vi "_nevstop_choosingDlg.vi"(8 "error in (no error)":errorcluster) -> (0 "error out":errorcluster, 1 "Cancelled?":bool=TRUE, 2 "QuckDrop":string, 3 "QDKS Info":T2[](array[typedef])=[{"VI Name"="Cluster AutoSizing", "VI Path"=path "C:/Program Files (x86)/National Instruments/LabVIEW 2014/resource/dialog/QuickDrop/plugins/QD_Cluster AutoSizing/Cluster AutoSizing.vi", "Default Shortcut"="U", "Assigned Shortcut"="u", "Description"="Using a float dialog to choose cluster auto-sizing type. Press `Shift` to set the contained cluster items recursively. \n\n- None\n- Size to Fit\n- Arrange Horizontally\n- Arrange Vertically\n\nDefault Shortcut - [U]"}, {"VI Name"="Align - Bottom Edges", "VI Path"=path "C:/Program Files (x86)/National Instruments/LabVIEW 2014/resource/dialog/QuickDrop/plugins/QD_Align&Distribute/Align - Bottom Edges.vi", "Default Shortcut"="v", "Assigned Shortcut"="v", "Description"="Align - Bottom Edges.vi\n"}, {"VI Name"="Align - Horizontal Centers", "VI Path"=path "C:/Program Files (x86)/National Instruments/LabVIEW 2014/resource/dialog/QuickDrop/plugins/QD_Align&Distribute/Align - Horizontal Centers.vi", "Default Shortcut"="v", "Assigned Shortcut"="", "Description"="Align - Horizontal Centers.vi"}, {"VI Name"="Align - Left Edges", "VI Path"=path "C:/Program Files (x86)/National Instruments/LabVIEW 2014/resource/dialog/QuickDrop/plugins/QD_Align&Distribute/Align - Left Edges.vi", "Default Shortcut"="v", "Assigned Shortcut"="5", "Description"="Align - Left Edges.vi"}, {"VI Name"="Align - Right Edges", "VI Path"=path "C:/Program Files (x86)/National Instruments/LabVIEW 2014/resource/dialog/QuickDrop/plugins/QD_Align&Distribute/Align - Right Edges.vi", "Default Shortcut"="v", "Assigned Shortcut"="", "Description"="Align - Right Edges.vi"}, {"VI Name"="Align - Top Edges", "VI Path"=path "C:/Program Files (x86)/National Instruments/LabVIEW 2014/resource/dialog/QuickDrop/plugins/QD_Align&Distribute/Align - Top Edges.vi", "Default Shortcut"="v", "Assigned Shortcut"="", "Description"="Align - Top Edges.vi"}, {"VI Name"="Align - Vertical Centers", "VI Path"=path "C:/Program Files (x86)/National Instruments/LabVIEW 2014/resource/dialog/QuickDrop/plugins/QD_Align&Distribute/Align - Vertical Centers.vi", "Default Shortcut"="v", "Assigned Shortcut"="", "Description"="Align - Vertical Centers.vi"}, {"VI Name"="Align and Distribute", "VI Path"=path "C:/Program Files (x86)/National Instruments/LabVIEW 2014/resource/dialog/QuickDrop/plugins/QD_Align&Distribute/Align and Distribute.vi", "Default Shortcut"="A", "Assigned Shortcut"="a", "Description"="Aligns selected items to the right, left, top or bottom or by horizontal or vertical centers by pressing r, l, t, b, h or v."}, {"VI Name"="Arrange VI Window", "VI Path"=path "C:/Program Files (x86)/National Instruments/LabVIEW 2014/resource/dialog/QuickDrop/plugins/QD_Arrange VI Window/Arrange VI Window.vi", "Default Shortcut"="F", "Assigned Shortcut"="f", "Description"="When used on the front panel:\n-Arranges controls and indicators to be consistent with the connector pane arrangement. \n-Resizes and moves the front panel to a consistent top left location on the primary monitor.\n\nWhen used on the block diagram:\n-Scrolls the block diagram to a reasonable location relative to the top-most and/or left-most diagram object.\n-Resizes and moves the block diagram to a consistent top left location on the primary monitor.\n\nDefault Shortcut - [F]"}, {"VI Name"="Build Array of References", "VI Path"=path "C:/Program Files (x86)/National Instruments/LabVIEW 2014/resource/dialog/QuickDrop/plugins/QD_Build Array of References/Build Array of References_NEVSTOP.vi", "Default Shortcut"="B", "Assigned Shortcut"="b", "Description"="### Build Array of Reference/Build Cluster of Reference\n\nCreate references with 'Build Array'/'buddle' together.\n\nDefault Shortcut - [B]"}, {"VI Name"="Build Cluster Of Reference", "VI Path"=path "C:/Program Files (x86)/National Instruments/LabVIEW 2014/resource/dialog/QuickDrop/plugins/QD_Build Cluster of References/Build Cluster Of Reference.vi", "Default Shortcut"="$", "Assigned Shortcut"="2", "Description"="Write a 1-2 sentence description of the functionality of your plugin here.  Replace the \"$\" below with the character you wish to assign as the default shortcut for this plugin.  Do not add any text after the 'Default Shortcut' line below.\n\nDefault Shortcut - [$]"}, {"VI Name"="Clone Control", "VI Path"=path "C:/Program Files (x86)/National Instruments/LabVIEW 2014/resource/dialog/QuickDrop/plugins/QD_Clone Control/Clone Control.vi", "Default Shortcut"="", "Assigned Shortcut"="", "Description"="Clones the selected Control(s) or Indicator(s) on the Front Panel but changes Controls to Indicators and vice versa.  In addition, if found on the Connector Pane, will attempt to place the newly created control on the opposite (left / right) side of the Connector Pane.\nNote: This script only supports the following patterns: 4x2x2x4, 5x3x3x5, 6x4x4x6, and 8x6x6x8.\n\nDefault Shortcut - [A]"}, {"VI Name"="Cluster AutoSizing - Arrange Horizontally", "VI Path"=path "C:/Program Files (x86)/National Instruments/LabVIEW 2014/resource/dialog/QuickDrop/plugins/QD_Cluster AutoSizing/Cluster AutoSizing - Arrange Horizontally.vi", "Default Shortcut"="v", "Assigned Shortcut"="", "Description"="Cluster AutoSizing - Arrange Horizontally.vi"}, {"VI Name"="Cluster AutoSizing - Arrange Veritcally", "VI Path"=path "C:/Program Files (x86)/National Instruments/LabVIEW 2014/resource/dialog/QuickDrop/plugins/QD_Cluster AutoSizing/Cluster AutoSizing - Arrange Veritcally.vi", "Default Shortcut"="v", "Assigned Shortcut"="", "Description"="Cluster AutoSizing - Arrange Veritcally.vi"}, {"VI Name"="Cluster AutoSizing - None", "VI Path"=path "C:/Program Files (x86)/National Instruments/LabVIEW 2014/resource/dialog/QuickDrop/plugins/QD_Cluster AutoSizing/Cluster AutoSizing - None.vi", "Default Shortcut"="v", "Assigned Shortcut"="", "Description"="Cluster AutoSizing - None.vi"}, {"VI Name"="Cluster AutoSizing - Size to Fit", "VI Path"=path "C:/Program Files (x86)/National Instruments/LabVIEW 2014/resource/dialog/QuickDrop/plugins/QD_Cluster AutoSizing/Cluster AutoSizing - Size to Fit.vi", "Default Shortcut"="v", "Assigned Shortcut"="", "Description"="Cluster AutoSizing - Size to Fit.vi"}, {"VI Name"="ColourUpStructures", "VI Path"=path "C:/Program Files (x86)/National Instruments/LabVIEW 2014/resource/dialog/QuickDrop/plugins/QD_ColourUpStructures/ColourUpStructures.vi", "Default Shortcut"="s", "Assigned Shortcut"="s", "Description"="Colour Up Structures."}, {"VI Name"="Copy Boolean Caption to BooleanText", "VI Path"=path "C:/Program Files (x86)/National Instruments/LabVIEW 2014/resource/dialog/QuickDrop/plugins/QD_Controls Operation/Copy Boolean Caption to BooleanText.vi", "Default Shortcut"="d", "Assigned Shortcut"="", "Description"="Copy selected boolean's caption to boolean text. If the booleans have no caption, label Text will be used instead."}, {"VI Name"="Create a Place VI Contents", "VI Path"=path "C:/Program Files (x86)/National Instruments/LabVIEW 2014/resource/dialog/QuickDrop/plugins/QD_Create a Place VI Contents/Create a Place VI Contents.vi", "Default Shortcut"="G", "Assigned Shortcut"="g", "Description"="(Note: The following shortcut was originally posted by Jarrod S. on the NI Forums here.  I decided to give his shortcut a more permanent home in the Quick Drop Enthusiasts group.)\n \nThis Quick Drop Keyboard Shortcut allows you to create a Place VI Contents VI (formerly called a \"Merge VI\") of your diagram selection and automatically create a user.lib palette entry for it, so that you can easily drop that selection of code in the future.  Follow these steps to use this shortcut:\n \nSave the attached VI in your <LabVIEW>\\resource\\dialog\\QuickDrop\\plugins folder.  No LabVIEW restart is required.\nSelect something on your diagram that you wish to make into a Place VI Contents VI.\nPress Ctrl-Space-Ctrl-Shift-G.\nSpecify a name for this Place VI Contents VI.\nCreate an icon\n \nNow you have a Place VI Contents VI that contains this diagram selection that you can use from your palettes (or Quick Drop).  Note that in step (3) above, if you had pressed Ctrl-Space-Ctrl-G instead, the palettes would not be refreshed automatically, and you would have to restart LabVIEW in order to use the new Place VI Contents VI.\n \nNote:  All Place VI Contents VIs that are created with this shortcut are stored in <LabVIEW Data>\\QuickDrop Templates.  The actual .mnu files that provide the palette entries are stored in <LabVIEW>\\user.lib\\QuickDrop Templates Palette.mnu.\n\n\nDefault Shortcut - [G]"}, {"VI Name"="Disable Controls", "VI Path"=path "C:/Program Files (x86)/National Instruments/LabVIEW 2014/resource/dialog/QuickDrop/plugins/QD_Controls Operation/Disable Controls.vi", "Default Shortcut"="l", "Assigned Shortcut"="l", "Description"="Disable Controls"}, {"VI Name"="Disable&Grayout Controls", "VI Path"=path "C:/Program Files (x86)/National Instruments/LabVIEW 2014/resource/dialog/QuickDrop/plugins/QD_Controls Operation/Disable&Grayout Controls.vi", "Default Shortcut"="l", "Assigned Shortcut"="", "Description"="Disable and grayout Controls"}, {"VI Name"="Distribute - Bottom Edges", "VI Path"=path "C:/Program Files (x86)/National Instruments/LabVIEW 2014/resource/dialog/QuickDrop/plugins/QD_Align&Distribute/Distribute - Bottom Edges.vi", "Default Shortcut"="v", "Assigned Shortcut"="", "Description"="Distribute - Bottom Edges.vi"}, {"VI Name"="Distribute - Horizontal Centers", "VI Path"=path "C:/Program Files (x86)/National Instruments/LabVIEW 2014/resource/dialog/QuickDrop/plugins/QD_Align&Distribute/Distribute - Horizontal Centers.vi", "Default Shortcut"="v", "Assigned Shortcut"="", "Description"="Distribute - Horizontal Centers.vi"}, {"VI Name"="Distribute - Horizontal Compress", "VI Path"=path "C:/Program Files (x86)/National Instruments/LabVIEW 2014/resource/dialog/QuickDrop/plugins/QD_Align&Distribute/Distribute - Horizontal Compress.vi", "Default Shortcut"="v", "Assigned Shortcut"="", "Description"="Distribute - Horizontal Compress.vi"}, {"VI Name"="Distribute - Horizontal Gap", "VI Path"=path "C:/Program Files (x86)/National Instruments/LabVIEW 2014/resource/dialog/QuickDrop/plugins/QD_Align&Distribute/Distribute - Horizontal Gap.vi", "Default Shortcut"="v", "Assigned Shortcut"="", "Description"="Distribute - Horizontal Gap.vi"}, {"VI Name"="Distribute - Left Edges", "VI Path"=path "C:/Program Files (x86)/National Instruments/LabVIEW 2014/resource/dialog/QuickDrop/plugins/QD_Align&Distribute/Distribute - Left Edges.vi", "Default Shortcut"="v", "Assigned Shortcut"="", "Description"="Distribute - Left Edges.vi"}, {"VI Name"="Distribute - Right Edges", "VI Path"=path "C:/Program Files (x86)/National Instruments/LabVIEW 2014/resource/dialog/QuickDrop/plugins/QD_Align&Distribute/Distribute - Right Edges.vi", "Default Shortcut"="v", "Assigned Shortcut"="", "Description"="Distribute - Right Edges.vi"}, {"VI Name"="Distribute - Top Edges", "VI Path"=path "C:/Program Files (x86)/National Instruments/LabVIEW 2014/resource/dialog/QuickDrop/plugins/QD_Align&Distribute/Distribute - Top Edges.vi", "Default Shortcut"="v", "Assigned Shortcut"="", "Description"="Distribute - Top Edges.vi"}, {"VI Name"="Distribute - Vertical Centers", "VI Path"=path "C:/Program Files (x86)/National Instruments/LabVIEW 2014/resource/dialog/QuickDrop/plugins/QD_Align&Distribute/Distribute - Vertical Centers.vi", "Default Shortcut"="v", "Assigned Shortcut"="", "Description"="Distribute - Vertical Centers.vi"}, {"VI Name"="Distribute - Vertical Compress", "VI Path"=path "C:/Program Files (x86)/National Instruments/LabVIEW 2014/resource/dialog/QuickDrop/plugins/QD_Align&Distribute/Distribute - Vertical Compress.vi", "Default Shortcut"="v", "Assigned Shortcut"="", "Description"="Distribute - Vertical Compress.vi"}, {"VI Name"="Distribute - Vertical Gap", "VI Path"=path "C:/Program Files (x86)/National Instruments/LabVIEW 2014/resource/dialog/QuickDrop/plugins/QD_Align&Distribute/Distribute - Vertical Gap.vi", "Default Shortcut"="v", "Assigned Shortcut"="", "Description"="Distribute - Vertical Gap.vi"}, {"VI Name"="EasyConvert", "VI Path"=path "C:/Program Files (x86)/National Instruments/LabVIEW 2014/resource/dialog/QuickDrop/plugins/EasyConvert.vi", "Default Shortcut"="e", "Assigned Shortcut"="7", "Description"="Typecast or convert a constant/control/VI/terminal into another. Will use other palette objects like U8 to String if the type string matches.\n\nHold shift while using Cntrl-E to always use the Typecase with constant instead of selecting based on the coded algorithm.\n\nDefault Shortcut - [e]"}, {"VI Name"="Enable Controls", "VI Path"=path "C:/Program Files (x86)/National Instruments/LabVIEW 2014/resource/dialog/QuickDrop/plugins/QD_Controls Operation/Enable Controls.vi", "Default Shortcut"="l", "Assigned Shortcut"="", "Description"="Enable Controls"}, {"VI Name"="Erease Data(Clear Data)", "VI Path"=path "C:/Program Files (x86)/National Instruments/LabVIEW 2014/resource/dialog/QuickDrop/plugins/QD_Erease Data/Erease Data(Clear Data).vi", "Default Shortcut"="E", "Assigned Shortcut"="e", "Description"="Clear control/Constant's data. Supported type:\n- Array\n- String\n- Listbox\n- MulticolumnListBox\n- Numeric\n- Table\n- Tree\n\nDefault Shortcut - [E]"}, {"VI Name"="Front Panel Clean-Up", "VI Path"=path "C:/Program Files (x86)/National Instruments/LabVIEW 2014/resource/dialog/QuickDrop/plugins/LMH-Toolbox/Front Panel Clean-Up.vi", "Default Shortcut"="$", "Assigned Shortcut"="4", "Description"="Write a 1-2 sentence description of the functionality of your plugin here.  Replace the \"$\" below with the character you wish to assign as the default shortcut for this plugin.  Do not add any text after the 'Default Shortcut' line below.\n\nDefault Shortcut - [$]"}, {"VI Name"="Hide Controls", "VI Path"=path "C:/Program Files (x86)/National Instruments/LabVIEW 2014/resource/dialog/QuickDrop/plugins/QD_Controls Operation/Hide Controls.vi", "Default Shortcut"="l", "Assigned Shortcut"="", "Description"="Hide Controls"}, {"VI Name"="Insert", "VI Path"=path "C:/Program Files (x86)/National Instruments/LabVIEW 2014/resource/dialog/QuickDrop/plugins/Insert.vi", "Default Shortcut"="I", "Assigned Shortcut"="i", "Description"="Inserts the object specified by name in the Quick Drop dialog box on the selected wire(s) on the diagram.  If [Shift] is also pressed, and multiple wires were selected, a single instance of the object is inserted on those wires.\n\nDefault Shortcut - [I]"}, {"VI Name"="JKI State Machine Helper", "VI Path"=path "C:/Program Files (x86)/National Instruments/LabVIEW 2014/resource/dialog/QuickDrop/plugins/JKI State Machine Helper__JKI_State_Machine_Helper.vi", "Default Shortcut"="j", "Assigned Shortcut"="j", "Description"="Launches JKI State Machine Helper.\n\nDefault Shortcut - [j]"}, {"VI Name"="Magic Delay Fairy", "VI Path"=path "C:/Program Files (x86)/National Instruments/LabVIEW 2014/resource/dialog/QuickDrop/plugins/Magic Delay Fairy/Magic Delay Fairy.vi", "Default Shortcut"="F", "Assigned Shortcut"="1", "Description"="Inserts a wait millisecond delay into selected error wires.\n\nDefault Shortcut - [F]"}, {"VI Name"="Move Labels", "VI Path"=path "C:/Program Files (x86)/National Instruments/LabVIEW 2014/resource/dialog/QuickDrop/plugins/Move Labels.vi", "Default Shortcut"="T", "Assigned Shortcut"="t", "Description"="Repositions the visible labels or captions of top-level front panel and block diagram objects to be consistent with the \"Default label position\" settings in Tools > Options. If [Shift] is also pressed, then all objects, including nested objects, are modified. If this shortcut is activated from the front panel, then controls and indicators are modified. If it is activated from the block diagram, then control and indicator terminals are modified. If panel or diagram objects were already selected when this shortcut is activated, only the selected objects that have visible labels or captions are modified.\n\nThe text justification of the modified labels and captions is also modified to be consistent with the new label or caption position.\n\nDefault Shortcut - [T]"}, {"VI Name"="NEVSTOP QD Shortcuts", "VI Path"=path "C:/Program Files (x86)/National Instruments/LabVIEW 2014/resource/dialog/QuickDrop/plugins/QD_NEVSTOP QD Shortcuts/NEVSTOP QD Shortcuts.vi", "Default Shortcut"="Q", "Assigned Shortcut"="q", "Description"="NEVSTOP Quickdrops. Using a choosing dialog for quick QD selection.\n\nDefault Shortcut - [Q]"}, {"VI Name"="Open Current VI Location in Explorer Window", "VI Path"=path "C:/Program Files (x86)/National Instruments/LabVIEW 2014/resource/dialog/QuickDrop/plugins/QD_Smart Open VI Location/Open Current VI Location.vi", "Default Shortcut"="w", "Assigned Shortcut"="", "Description"="Open Current VI Location in Explorer Window."}, {"VI Name"="Open Selected VI's Location in Explorer Window", "VI Path"=path "C:/Program Files (x86)/National Instruments/LabVIEW 2014/resource/dialog/QuickDrop/plugins/QD_Smart Open VI Location/Open Selected VI Location.vi", "Default Shortcut"="w", "Assigned Shortcut"="", "Description"="Open Selected VI's Location in Explorer Window."}, {"VI Name"="Refresh Palette", "VI Path"=path "C:/Program Files (x86)/National Instruments/LabVIEW 2014/resource/dialog/QuickDrop/plugins/QD_Create a Place VI Contents/Refresh Palette.vi", "Default Shortcut"="p", "Assigned Shortcut"="", "Description"="After some chane of Control/Function Pallette, you can manually update the pallette with this quickdrop.\n"}, {"VI Name"="Remove and Rewire", "VI Path"=path "C:/Program Files (x86)/National Instruments/LabVIEW 2014/resource/dialog/QuickDrop/plugins/Remove and Rewire.vi", "Default Shortcut"="R", "Assigned Shortcut"="r", "Description"="Removes the selected block diagram object(s) and any wires and constants connected to the selected object(s), and connects wires of identical data types that were wired to the inputs and outputs of the deleted object(s).\n\nDefault Shortcut - [R]"}, {"VI Name"="Replace", "VI Path"=path "C:/Program Files (x86)/National Instruments/LabVIEW 2014/resource/dialog/QuickDrop/plugins/Replace.vi", "Default Shortcut"="P", "Assigned Shortcut"="p", "Description"="Replaces the selected panel or diagram object(s) with the object specified by name in the Quick Drop dialog box.\n\nDefault Shortcut - [P]"}, {"VI Name"="Reset Origin", "VI Path"=path "C:/Program Files (x86)/National Instruments/LabVIEW 2014/resource/dialog/QuickDrop/plugins/QD_Controls Operation/Reset Origin.vi", "Default Shortcut"=")", "Assigned Shortcut"=")", "Description"="Reset the origin of the front panel or block diagram to (0,0).\n"}, {"VI Name"="Show Controls", "VI Path"=path "C:/Program Files (x86)/National Instruments/LabVIEW 2014/resource/dialog/QuickDrop/plugins/QD_Controls Operation/Show Controls.vi", "Default Shortcut"="l", "Assigned Shortcut"="", "Description"="Show Controls"}, {"VI Name"="Smart Open VI Locaiton in Explorer Window", "VI Path"=path "C:/Program Files (x86)/National Instruments/LabVIEW 2014/resource/dialog/QuickDrop/plugins/QD_Smart Open VI Location/Smart Open VI Locaiton.vi", "Default Shortcut"="O", "Assigned Shortcut"="o", "Description"="When triggered on Front Panel:\nOpen Current VI's Location in Explorer Window.\n\nWhen triggered on Block Diagram:\nNo SubVI is selected: Open Current VI's Location in Explorer Window.\nSubVIs are selected: Open Selected VI's Location in Explorer Window.\n\nDefault Shortcut - [O]"}, {"VI Name"="State Machine from Enum", "VI Path"=path "C:/Program Files (x86)/National Instruments/LabVIEW 2014/resource/dialog/QuickDrop/plugins/QD_State Machine From Enum/_old version/State Machine from Enum (2010).vi", "Default Shortcut"="s", "Assigned Shortcut"="", "Description"="Creates a state machine from a selected enum."}, {"VI Name"="Toggle Digital Increment Decrement Visible ( Swithc Show Or Hide )", "VI Path"=path "C:/Program Files (x86)/National Instruments/LabVIEW 2014/resource/dialog/QuickDrop/plugins/QD_Controls Operation/Toggle Digital Increment Decrement Visible ( Swithc Show Or Hide ).vi", "Default Shortcut"="v", "Assigned Shortcut"="", "Description"="Toggle Digital Increment Decrement Visible ( Swithc Show Or Hide ).vi"}, {"VI Name"="VI Server Rename", "VI Path"=path "C:/Program Files (x86)/National Instruments/LabVIEW 2014/resource/dialog/QuickDrop/plugins/VI Server Rename.vi", "Default Shortcut"="B", "Assigned Shortcut"="0", "Description"="Changes the VI Server class of the selected property node(s), invoke node(s), and/or Class Specifier Constants, to the class typed in the Quick Drop window.  If [Shift] is also pressed, changes the property/method of the selected property node(s)/invoke node(s), respectively, to the property/method name typed in the Quick Drop window.\n\nDefault Shortcut - [B]"}, {"VI Name"="While Loop Subdiagram Label", "VI Path"=path "C:/Program Files (x86)/National Instruments/LabVIEW 2014/resource/dialog/QuickDrop/plugins/QD_While Loop Subdiagram Label/While Loop Subdiagram Label.vi", "Default Shortcut"="r", "Assigned Shortcut"="", "Description"="Takes the text in the Quick Drop box and applies it as a subdiagram label to a While Loop, and formats the subdiagram label to have white, bold text, with the while loop's gray background color."}, {"VI Name"="Wire All Terminals", "VI Path"=path "C:/Program Files (x86)/National Instruments/LabVIEW 2014/resource/dialog/QuickDrop/plugins/Wire All Terminals.vi", "Default Shortcut"="D", "Assigned Shortcut"="d", "Description"="Creates controls and indicators for all unwired inputs and outputs of the selected block diagram object(s).  If 'shift' is also pressed, creates constants for all unwired inputs of the selected block diagram object(s).\n\nDefault Shortcut - [D]"}, {"VI Name"="Wire Multiple Objects Together", "VI Path"=path "C:/Program Files (x86)/National Instruments/LabVIEW 2014/resource/dialog/QuickDrop/plugins/Wire Multiple Objects Together.vi", "Default Shortcut"="W", "Assigned Shortcut"="w", "Description"="Connects compatible terminals between multiple selected diagram objects. This shortcut will wire compatible data types between the objects in a left-to-right fashion. If [Shift] is also pressed, LabVIEW will perform a diagram cleanup of the selected objects after wiring them together.\n\nDefault Shortcut - [W]"}], 4 "Shift Pressed":bool)   [LabVIEW 2020, in "NEVSTOP QD Shortcuts.lvlib"]
uses:
  NEVSTOP QD Shortcuts.lvlib
  <userlib>/_OpenG.lib/string/string.llb/Trim Whitespace (String)__ogtk.vi
  <userlib>/_OpenG.lib/file/file.llb/Compare Two Paths - Scalar__ogtk.vi
  <userlib>/_OpenG.lib/array/array.llb/Remove Duplicates from 1D Array (String)__ogtk.vi
  <resource>/dialog/QuickDrop/QuickDrop QDKS Info.ctl
  <vilib>/event_ctls.llb/eventvkey.ctl
panel:
  out "Path":path
  in  "[Trigger]Decorate List":bool=TRUE
  out "Variant":variant=variant("Align - Horizontal Centers"=variant(i32 2), "Align - Left Edges"=variant(i32 1), "Align and Distribute"=variant(i32 1), "Arrange VI Window"=variant(i32 1), "Build Array of References"=variant(i32 2), "Build Cluster Of Reference"=variant(i32 3), "Clone Control"=variant(i32 2), "Cluster AutoSizing"=variant(i32 4), "Cluster AutoSizing - None"=variant(i32 1), "Create a Place VI Contents"=variant(i32 1), "Distribute - Right Edges"=variant(i32 1), "Distribute - Vertical Compress"=variant(i32 1), "EasyConvert"=variant(i32 2), "Format Numeric"=variant(i32 1), "Front Panel Clean-Up"=variant(i32 4), "Move Labels"=variant(i32 1), "NEVSTOP QD Shortcuts"=variant(i32 1), "Show Controls"=variant(i32 1))
  in  "[Trigger]Update QSDK Info":bool=TRUE
  in  "[Trigger]Refresh Btns":bool=TRUE
  out "VKey":T1=enum."Escape"
  out "Info":string
  in  "FilterStr":string
  in  "Debug":bool
  out "Shift TEMP":bool
  in  "Shift":bool
  in  "M":bool caption="0"
  in  "N":bool caption="0"
  in  "L":bool caption="0"
  in  "K":bool caption="0"
  in  "J":bool caption="0"
  in  "H":bool caption="0"
  in  "P":bool caption="0"
  in  "O":bool caption="0"
  in  "I":bool caption="0"
  in  "U":bool caption="4"
  in  "Y":bool caption="0"
  in  "B":bool caption="2"
  in  "V":bool caption="0"
  in  "C":bool caption="0"
  in  "X":bool caption="0"
  in  "Z":bool caption="0"
  in  "G":bool caption="1"
  in  "F":bool caption="1"
  in  "D":bool caption="0"
  in  "S":bool caption="0"
  in  "A":bool caption="1"
  in  "T":bool caption="1"
  in  "R":bool caption="0"
  in  "E":bool caption="0"
  in  "W":bool caption="0"
  in  "Q":bool caption="1"
  in  "0":bool
  in  "9":bool caption="0"
  in  "8":bool caption="0"
  in  "7":bool caption="2"
  in  "6":bool caption="0"
  in  "5":bool caption="1"
  in  "4":bool
  in  "3":bool caption="0"
  in  "2":bool caption="3"
  in  "1":bool caption="0"
  in  "Listbox":i32(listbox)=-1
  out "Key Temp":string
  out "Char":i16
  # "Drag To Button, Change Assigned Shortcut, Drag to Shift, Clear Arrsigned Shortcut."
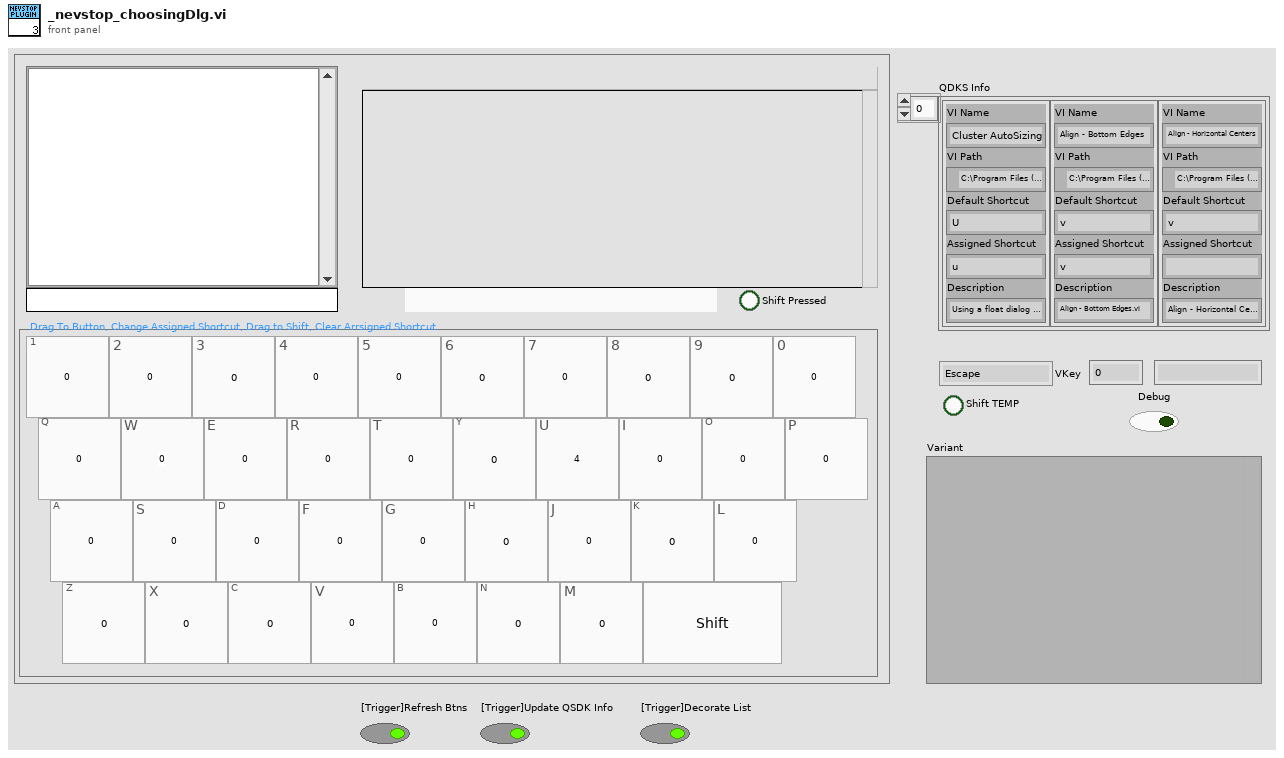
[diagram p1: front panel]
types:
  T1 = typedef "eventvkey.ctl" = enum16{"ASCII", "Enter", "Return", "Shift", "Ctrl", "Alt", "Cmd", "Opt", "Caps", "NumLock", "Clear", "Break", "Up", "Down", "Left", "Right", "Insert", "Delete", "Home", "End", "PageUp", "PageDown", "Escape", "Help", "Pause", "ScrollLock", "F1", "F2", "F3", "F4", "F5", "F6", "F7", "F8", "F9", "F10", "F11", "F12", "F13", "F14", "F15", "F16", "F17", "F18", "F19", "F20", "F21", "F22", "F23", "F24", "Play", "VolumeUp", "VolumeDown", "Mute", "Two Byte Char"}
  T2 = typedef "QuickDrop QDKS Info.ctl" = cluster{"VI Name":string, "VI Path":path, "Default Shortcut":string, "Assigned Shortcut":string, "Description":string}
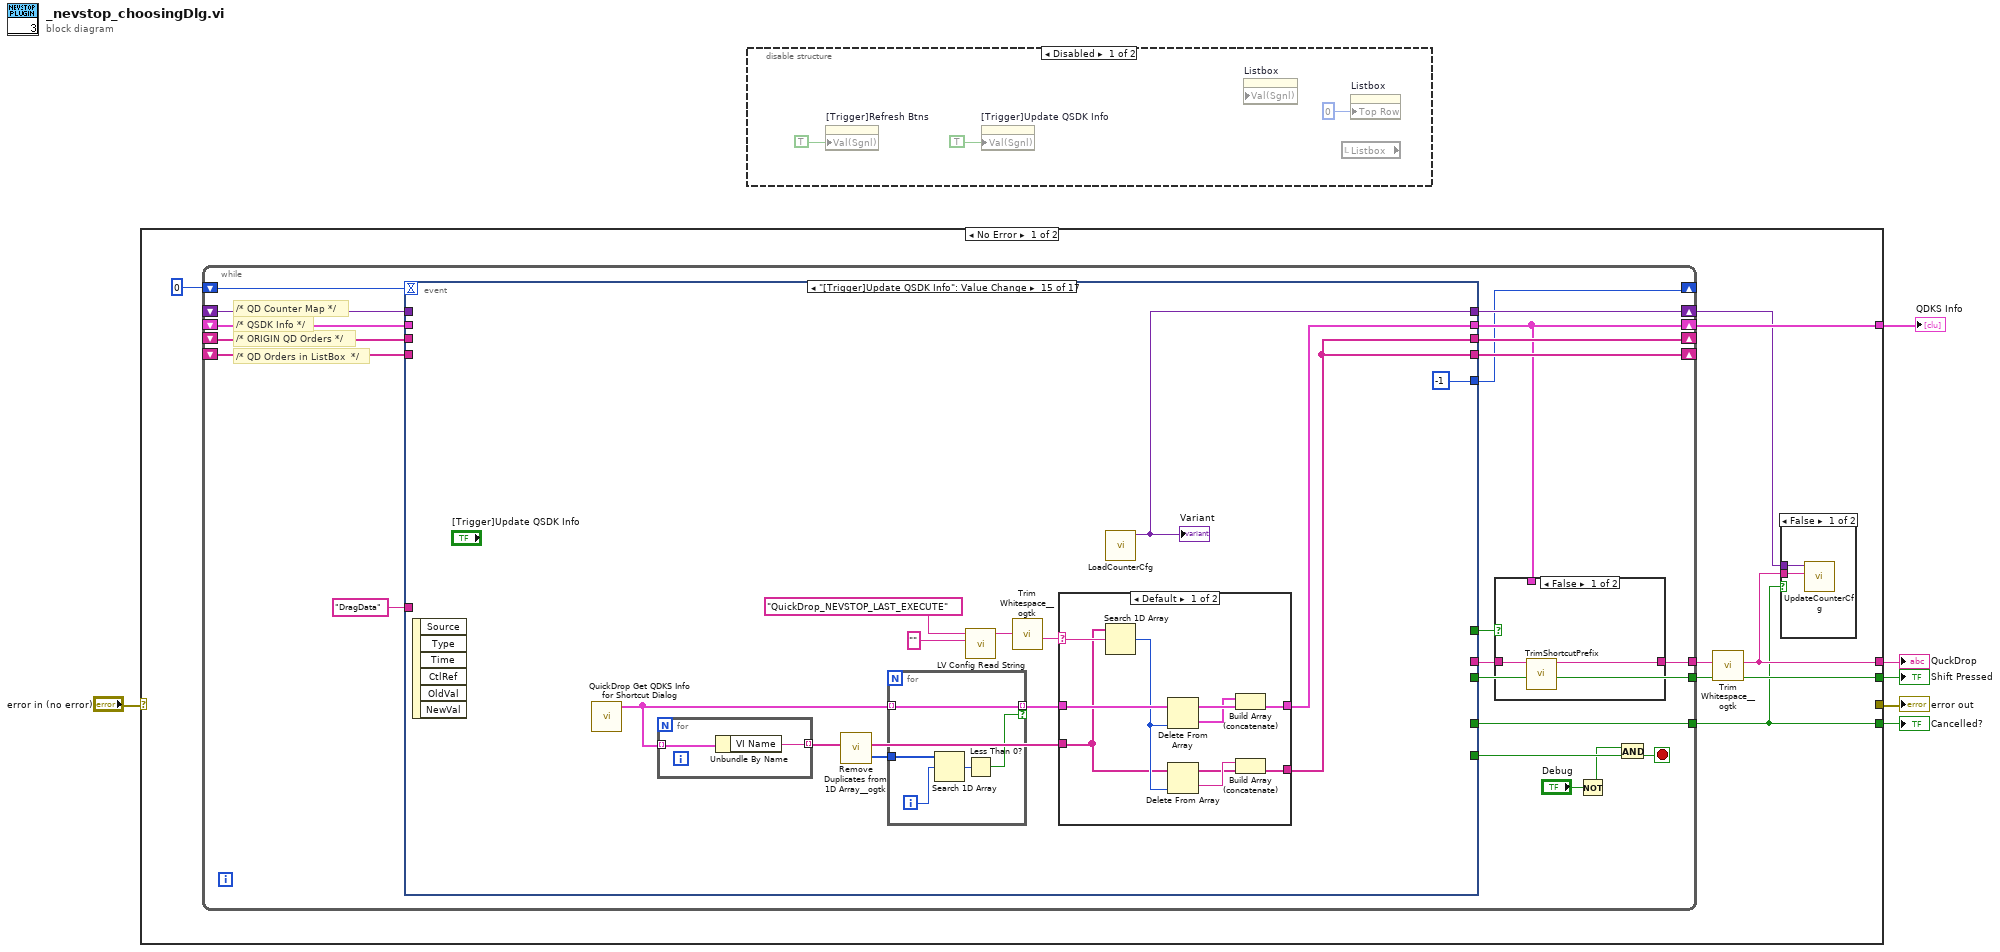
[diagram p0: block diagram]
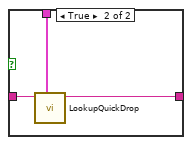
[diagram p4: hidden frame]
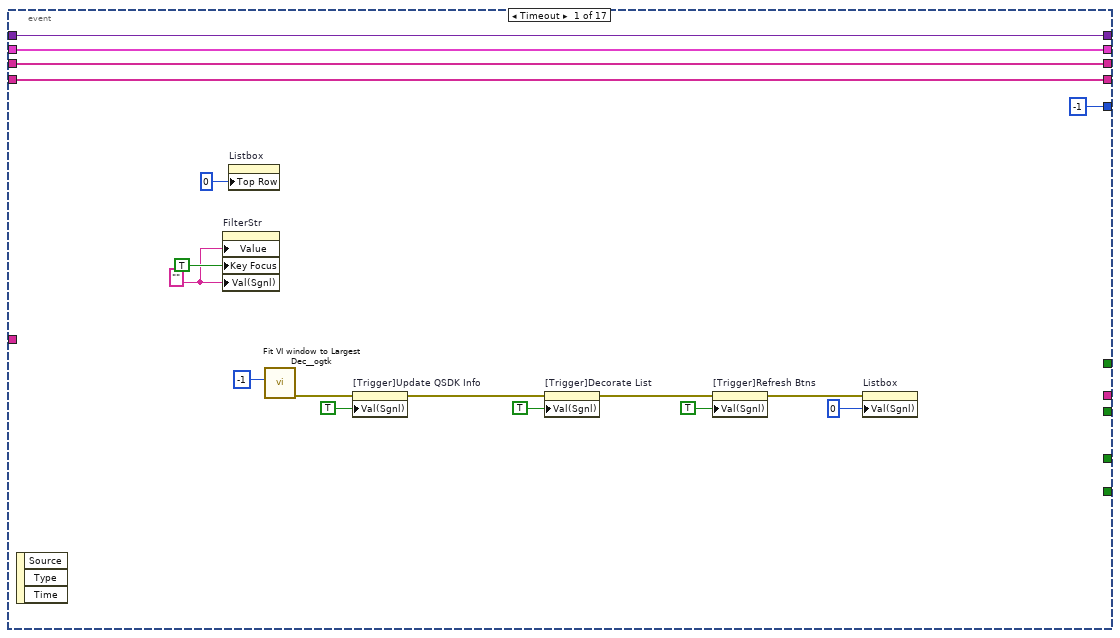
[diagram p5: hidden frame]
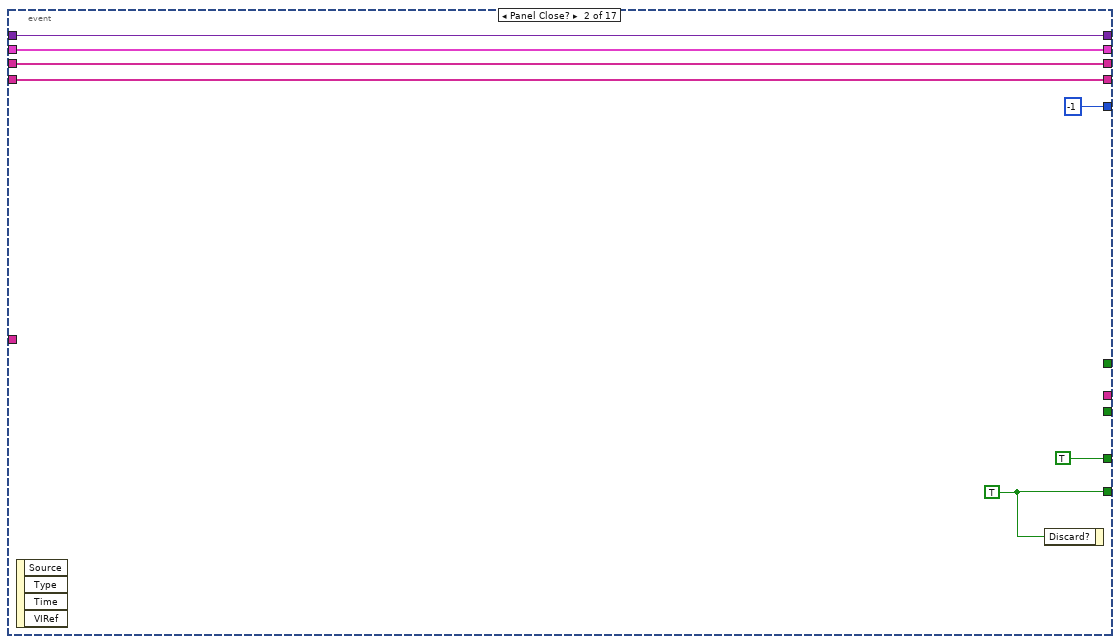
[diagram p6: hidden frame]
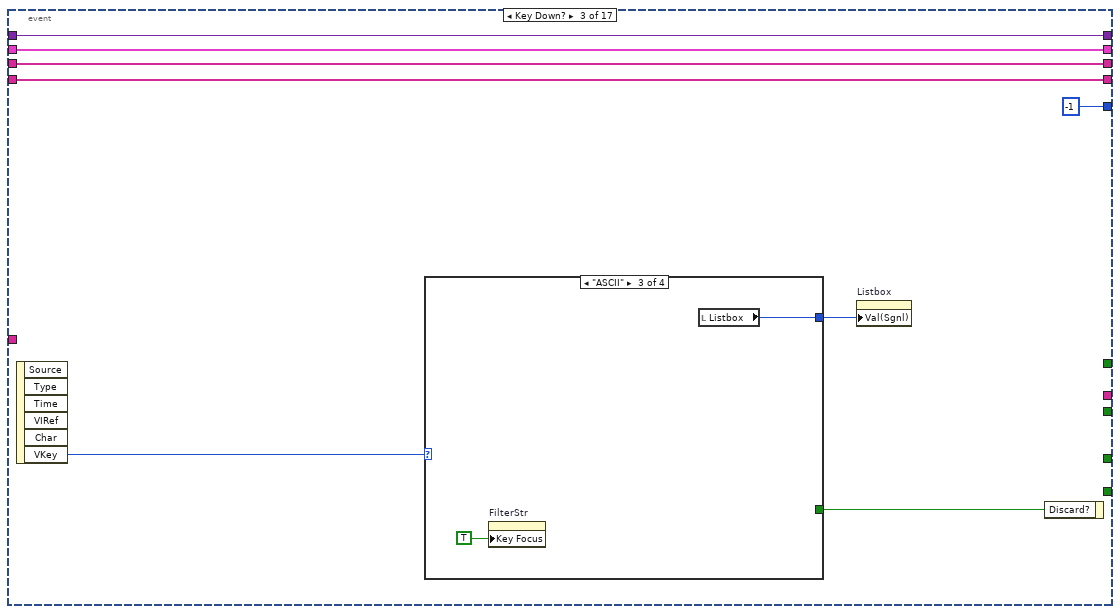
[diagram p7: hidden frame]
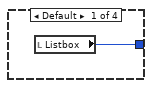
[diagram p8: hidden frame]
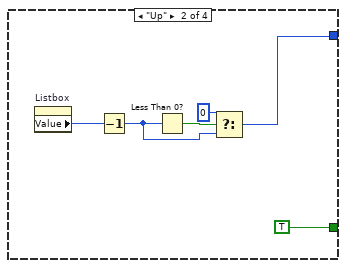
[diagram p9: hidden frame]
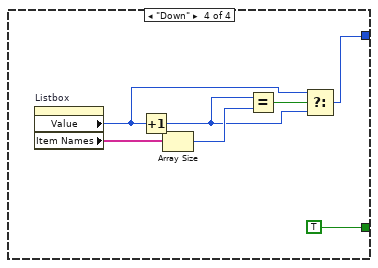
[diagram p10: hidden frame]
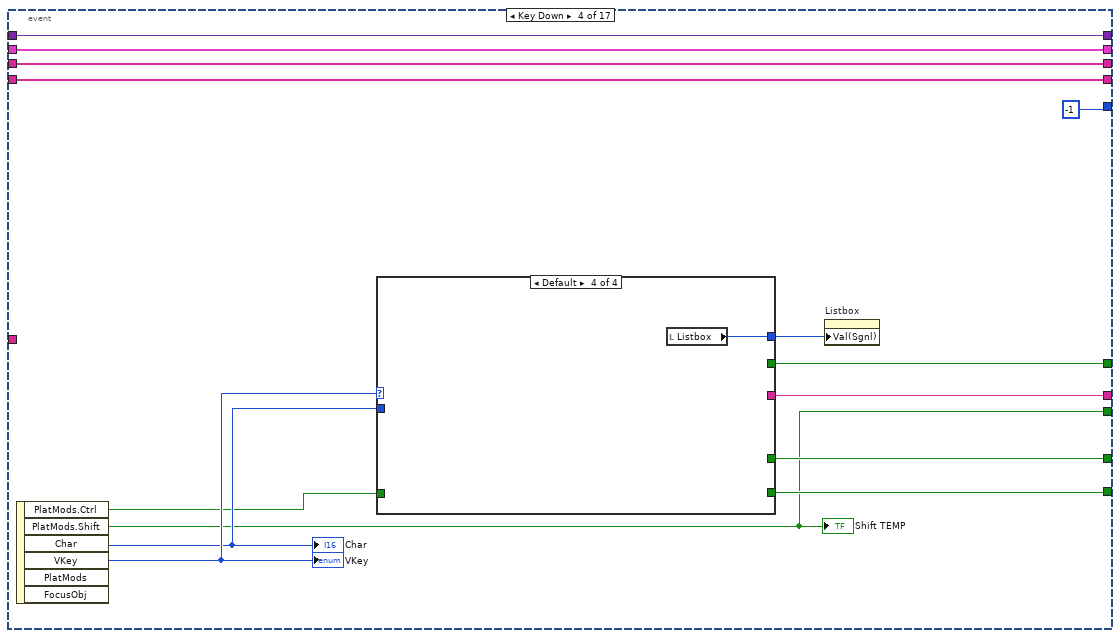
[diagram p11: hidden frame]
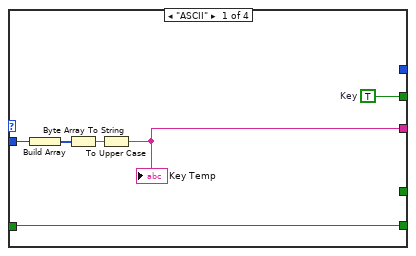
[diagram p12: hidden frame]
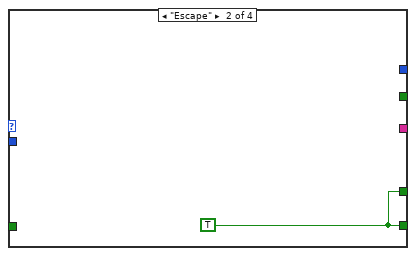
[diagram p13: hidden frame]
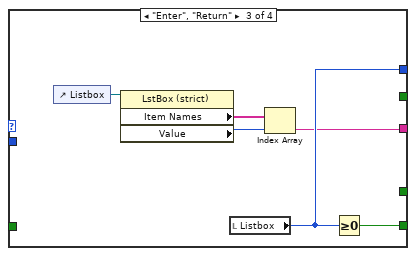
[diagram p14: hidden frame]
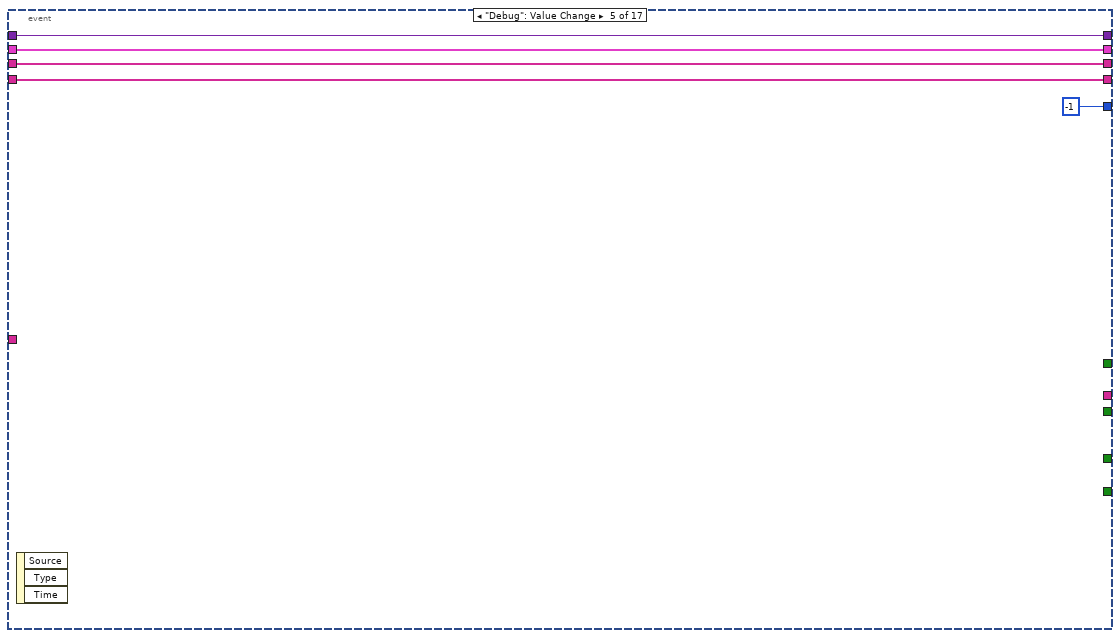
[diagram p15: hidden frame]
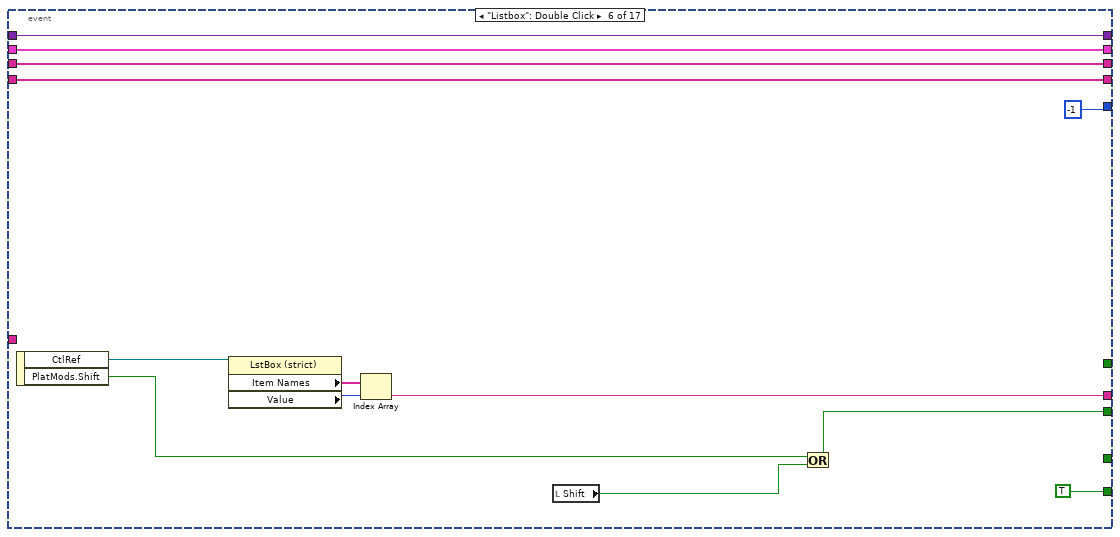
[diagram p16: hidden frame]
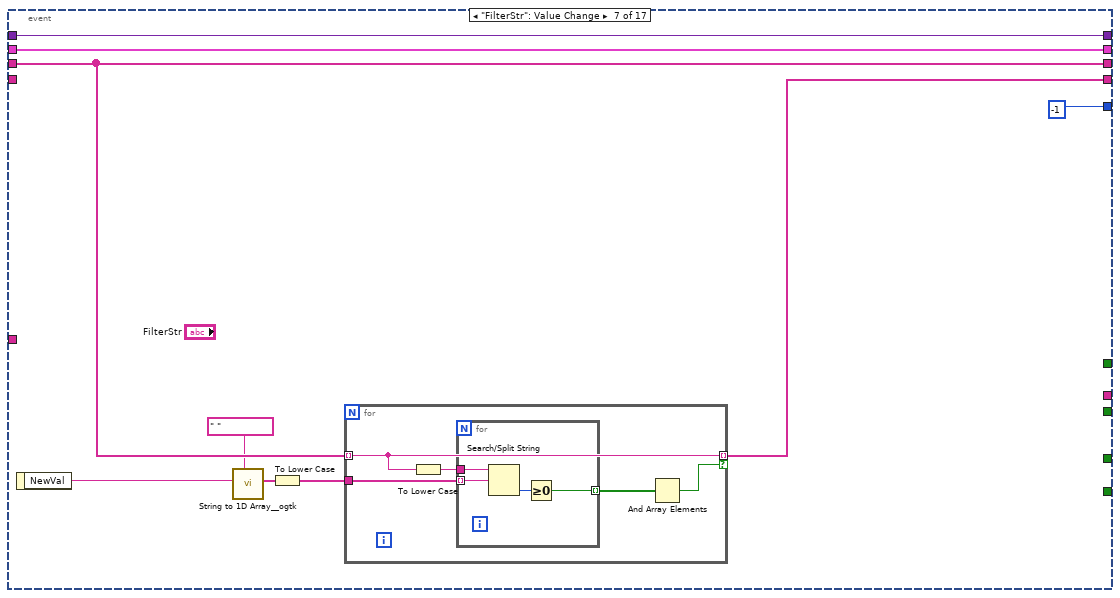
[diagram p17: hidden frame]
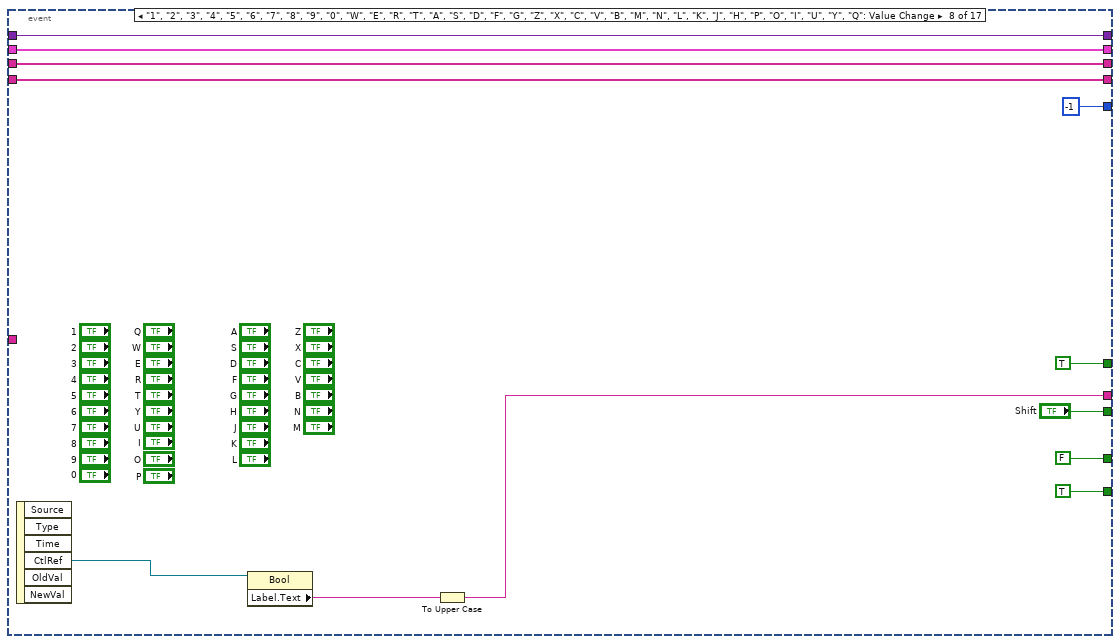
[diagram p18: hidden frame]
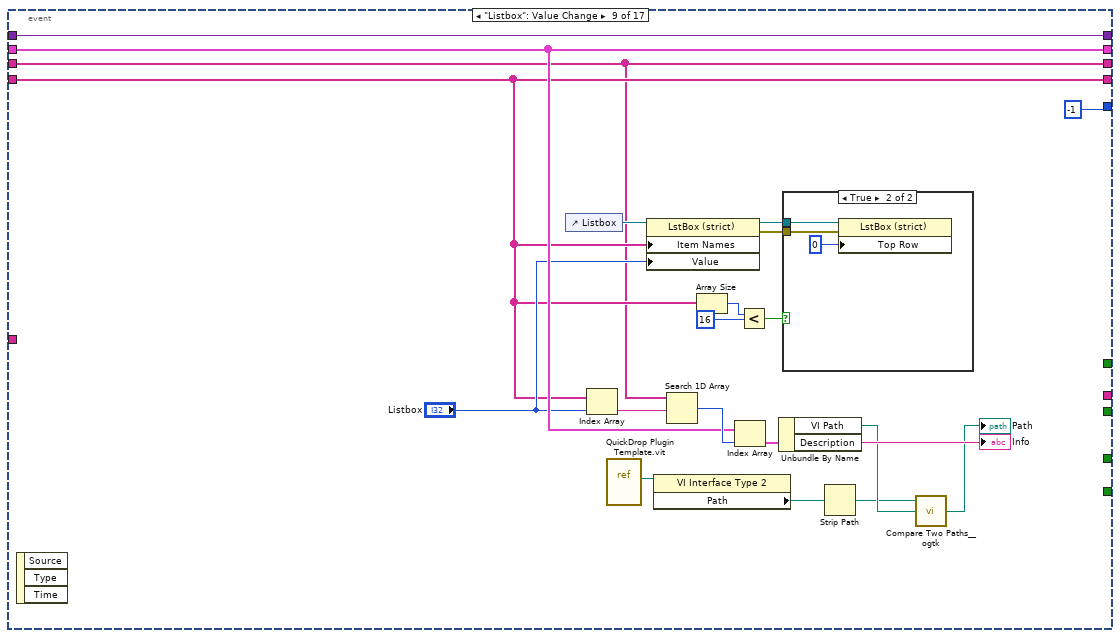
[diagram p19: hidden frame]
diagram:
  n1 = case shown="No Error" "error in (no error)" {
    selector: "error in (no error)" -> [_ w345]
    tunnel: [w7 TRUE] -> w6
    tunnel: [_ w345] -> w4
    tunnel: [w9 _] -> w3
    tunnel: [w11 _] -> w2
    tunnel: [w10 _] -> w1
    frame No Error {
      n2 = while {
        shift-right: [w16] -> _
        shift-left: 0 -> [w34]
        tunnel: [w33] -> w7
        tunnel: [w27] -> w12
        tunnel: [w32] -> w11
        shift-right: [w22] -> _
        shift-left: _ -> [w25]
        shift-right: [w17] -> w10
        shift-left: _ -> [w24]
        shift-right: [w20] -> _
        shift-left: _ -> [w23]
        shift-right: [w19] -> w8
        shift-left: _ -> [w18]
        stop <- w31 stop-if-true
        # "/* QD Orders in ListBox  */"
        # "/* ORIGIN QD Orders */"
        # "/* QD Counter Map */"
        # "/* QSDK Info */"
        n3 = event shown="[14] \"[Trigger]Update QSDK Info\": Value Change" {
          selector: _ -> [_ _ _ _ _ _ _ _ _ _ _ _ _ _ _ _ _]
          dyn-events: _ -> [_ _ _ _ _ _ _ _ _ _ _ _ _ _ _ _ _]
          timeout: w34 -> [_ _ _ _ _ _ _ _ _ _ _ _ _ _ _ _ _]
          tunnel: [_ w64 _ w99 _ TRUE ("Discard?") _ TRUE ("Discard?") _ _ _ _ _ _ _ _ _] -> w35
          tunnel: [_ TRUE _ w98 _ _ _ FALSE _ _ _ _ _ _ _ _ _] -> w33
          tunnel: [_ _ _ w100 _ w131 _ w160 _ _ _ _ _ _ _ _ _] -> w26
          tunnel: [_ _ _ w97 _ w129 _ "Shift" _ _ _ _ _ _ _ _ _] -> w32
          tunnel: [_ _ _ w94 _ _ _ TRUE ("Key") _ _ _ _ _ _ _ _ _] -> w28
          tunnel: w24 -> [w53 w61 w69 w93 w120 w125 w137 w156 w174 w192 w206 w225 w234 w256 _ w318 w323]
          tunnel: [w56 w62 w72 w96 w121 w127 w142 w157 w172 w202 w213 w230 w242 w273 w287 w319 w324] -> w22
          tunnel: w25 -> [w56 w62 w72 w96 w121 w127 _ w157 w172 w202 w213 w230 w242 w273 _ w319 _]
          tunnel: w23 -> [w52 w60 w68 w92 w119 w124 w143 w155 w171 w191 w205 w224 w233 w255 _ w317 _]
          tunnel: "DragData" -> [_ _ _ _ _ _ _ _ _ w195 w211 w228 w240 _ _ _ _]
          tunnel: [w53 w61 w69 w93 w120 w125 w137 w156 w174 w192 w206 w225 w234 w256 w288 w318 w323] -> w17
          tunnel: [w52 w60 w68 w92 w119 w124 w143 w155 w171 w191 w205 w224 w233 w255 w287 w317 w324] -> w20
          tunnel: [w49 w59 w67 w91 w118 w123 w136 w154 w185 w190 w204 w223 w232 w254 w286 w316 w320] -> w19
          tunnel: w18 -> [w49 w59 w67 w91 w118 w123 w136 w154 w185 w190 w204 w223 w232 w254 _ w316 w321]
          tunnel: [-1 -1 -1 -1 -1 -1 -1 -1 -1 -1 0 -1 0 -1 -1 -1 -1] -> w16
          event Timeout {
            w55 = "" ("Value (Signaling)")
            n4 = event-data() -> ()  [unwired: 1 in, 3 out]
            n5 = property on="FilterStr" class="Str"("Value"=w55, "Key Focus"=TRUE, "Val(Sgnl)"=w55) -> ()  [unwired: 2 in, 2 out]
            n6 = property on="Listbox" class="LstBox (strict)"("Top Row"=0) -> ()  [unwired: 2 in, 2 out]
            n7 = call <userlib>:"Fit VI window to Largest Dec__ogtk.vi"("border spacing (2 px)"=-1) -> ("error out"=w42:errorcluster)  [unwired: 5 in, 1 out]
            n8 = property on="[Trigger]Update QSDK Info" class="Bool (strict)"(error in=w42, "Val(Sgnl)"=TRUE ("Value (Signaling)")) -> (error out=w45:errorcluster)  [unwired: 1 in, 1 out]
            n9 = property on="[Trigger]Decorate List" class="Bool (strict)"(error in=w45, "Val(Sgnl)"=TRUE ("Value (Signaling)")) -> (error out=w44:errorcluster)  [unwired: 1 in, 1 out]
            n10 = property on="[Trigger]Refresh Btns" class="Bool (strict)"(error in=w44, "Val(Sgnl)"=TRUE ("Value (Signaling)")) -> (error out=w48:errorcluster)  [unwired: 1 in, 1 out]
            n11 = property on="Listbox" class="LstBox (strict)"(error in=w48, "Val(Sgnl)"=0) -> ()  [unwired: 1 in, 2 out]
          }
          event Panel Close? {
            w64 = TRUE ("Discard?")
            n12 = event-data() -> ()  [unwired: 1 in, 4 out]
            n13 = event-data("Discard?"=w64) -> ()  [unwired: 1 in, 1 out]
          }
          event Key Down? {
            n14 = event-data() -> ("VKey"=w71:T1)  [unwired: 1 in, 5 out]
            n15 = case shown="\"ASCII\"" w71 {
              tunnel: [_ TRUE _ TRUE] -> w70
              tunnel: [w73 w74 w81 w82] -> w66
              frame Default {
                n16 = local read "Listbox"() -> (w73:i32)
              }
              frame "Up" {
                n17 = property on="Listbox" class="LstBox (strict)"() -> ("Value"=w78:i32)  [unwired: 2 in, 2 out]
                n18 = Decrement(x=w78) -> (x-1=w75:i32)
                n19 = Less Than 0?(x=w75) -> (x < 0?=w77:bool)
                n20 = Select(t=0, s=w77, f=w75) -> (s? t:f=w74:i32)
              }
              frame "ASCII" {
                n21 = property on="FilterStr" class="Str"("Key Focus"=TRUE) -> ()  [unwired: 2 in, 2 out]
                n22 = local read "Listbox"() -> (w81:i32)
              }
              frame "Down" {
                n23 = property on="Listbox" class="LstBox (strict)"() -> ("Value"=w83:i32, "Item Names"=w87:string[])  [unwired: 2 in, 2 out]
                n24 = Increment(x=w83) -> (x+1=w84:i32)
                n25 = Array Size(array=w87) -> (size(s)=w86:i32)
                n26 = Equal?(x=w84, y=w86) -> (x = y?=w85:bool)
                n27 = Select(t=w83, s=w85, f=w84) -> (s? t:f=w82:i32)
              }
            }
            n28 = property on="Listbox" class="LstBox (strict)"("Val(Sgnl)"=w66) -> ()  [unwired: 2 in, 2 out]
            n29 = event-data("Discard?"=w70) -> ()  [unwired: 1 in, 1 out]
          }
          event Key Down {
            n30 = event-data() -> ("PlatMods.Ctrl"=w95:bool, "PlatMods.Shift"=w97:bool, "Char"=w101:i16, "VKey"=w102:T1)  [unwired: 1 in, 2 out]
            "Char" <- w101
            "Shift TEMP" <- w97
            "VKey" <- w102
            n31 = case shown="Default" w102 {
              tunnel: w101 -> [w108 _ _ _]
              tunnel: [w105 _ w110 _] -> w100
              tunnel: [w104 w109 w115 _] -> w99
              tunnel: [_ w109 _ _] -> w98
              tunnel: w95 -> [w104 _ _ _]
              tunnel: [w103 _ _ _] -> w94
              tunnel: [_ _ w114 w116] -> w90
              frame "ASCII" {
                w103 = TRUE  # Key
                n32 = Build Array(w108) -> (w107:i16[])
                n33 = Byte Array To String(unsigned byte array=w107) -> (string=w106:string)
                n34 = To Upper Case(1:w106) -> (0:w105:string)
                "Key Temp" <- w105
              }
              frame "Escape" {
                w109 = TRUE
              }
              frame "Enter", "Return" {
                n35 = control-ref of="Listbox"() -> (w113:refnum<vi>)
                n36 = property on="Property Node" class="LstBox (strict)"(reference=w113) -> ("Item Names"=w112:string[], "Value"=w111:i32)  [unwired: 1 in, 2 out]
                n37 = local read "Listbox"() -> (w114:i32)
                n38 = Index Array(array=w112, index=w111) -> (element=w110:string)
                n39 = Greater Or Equal To 0?(x=w114) -> (x >= 0?=w115:bool)
              }
              frame Default {
                n40 = local read "Listbox"() -> (w116:i32)
              }
            }
            n41 = property on="Listbox" class="LstBox (strict)"("Val(Sgnl)"=w90) -> ()  [unwired: 2 in, 2 out]
          }
          event "Debug": Value Change {
            n42 = event-data() -> ()  [unwired: 1 in, 3 out]
          }
          event "Listbox": Double Click {
            n43 = event-data() -> ("CtlRef"=w133:refnum<vi>, "PlatMods.Shift"=w128:bool)  [unwired: 1 in]
            n44 = property class="LstBox (strict)"(reference=w133) -> ("Item Names"=w132:string[], "Value"=w126:i32)  [unwired: 1 in, 2 out]
            n45 = Index Array(array=w132, index=w126) -> (element=w131:string)
            n46 = local read "Shift"() -> (w130:bool)
            n47 = Or(x=w128, y=w130) -> (x .or. y?=w129:bool)
          }
          event "FilterStr": Value Change {
            n48 = event-data() -> ("NewVal"=w140:string)  [unwired: 1 in]
            n49 = call <userlib>:"String to 1D Array__ogtk.vi"("delimiter (Tab)"=" ", "string"=w140) -> ("Array of Strings"=w141:string[])  [unwired: 9 in]
            n50 = To Lower Case(string=w141) -> (all lower case string=w139:string[])
            n51 = for {
              tunnel: w143 -> [w147] mode=indexing
              tunnel: w139 -> [w148]
              tunnel: [w147] -> w142 mode=indexing if=w144
              n52 = To Lower Case(string=w147) -> (all lower case string=w145:string)
              n53 = for {
                tunnel: [w151] -> w146 mode=indexing
                tunnel: w145 -> [w150]
                tunnel: w148 -> [w149] mode=indexing
                n54 = Search/Split String(string=w150, search string/char (-)=w149) -> (offset of match=w152:i32)  [unwired: 1 in, 2 out]
                n55 = Greater Or Equal To 0?(x=w152) -> (x >= 0?=w151:bool)
              }
              n56 = And Array Elements(Boolean array=w146) -> (logical AND=w144:bool)
            }
          }
          event "1", "2", "3", "4", "5", "6", "7", "8", "9", "0", "W", "E", "R", "T", "A", "S", "D", "F", "G", "Z", "X", "C", "V", "B", "M", "N", "L", "K", "J", "H", "P", "O", "I", "U", "Y", "Q": Value Change {
            n57 = event-data() -> ("CtlRef"=w164:refnum<vi>)  [unwired: 1 in, 5 out]
            n58 = property class="Bool"(reference=w164) -> ("Label.Text"=w163:string)  [unwired: 1 in, 2 out]
            n59 = To Upper Case(1:w163) -> (0:w160:string)
          }
          event "Listbox": Value Change {
            n60 = event-data() -> ()  [unwired: 1 in, 3 out]
            n61 = control-ref of="Listbox"() -> (w181:refnum<vi>)
            n62 = Index Array(array=w172, index="Listbox") -> (element=w178:string)
            n63 = vi-ref <resource>:"QuickDrop Plugin Template.vit"() -> (w169:refnum<vi>)
            n64 = property on="Property Node" class="LstBox (strict)"(reference=w181, "Item Names"=w172, "Value"="Listbox") -> (reference out=w180:refnum<vi>, error out=w179:errorcluster)  [unwired: 1 in]
            n65 = property class="VI Interface Type 2"(reference=w169) -> ("Path"=w168:path)  [unwired: 1 in, 2 out]
            n66 = Search 1D Array(1D array=w171, element=w178) -> (index of element=w175:i32)  [unwired: 1 in]
            n67 = Array Size(array=w172) -> (size(s)=w182:i32)
            n68 = Index Array(array=w174, index=w175) -> (element=w176:T2)
            n69 = Less?(x=w182, y=16) -> (x < y?=w184:bool)
            n70 = Unbundle By Name(w176) -> ("VI Path"=w167:path, "Description"=→"Info":string)
            n71 = case shown="True" w184 {
              tunnel: w179 -> [_ w188]
              tunnel: w180 -> [_ w187]
              frame False {
              }
              frame True {
                n72 = property on="Property Node" class="LstBox (strict)"(reference=w187, error in=w188, "Top Row"=0) -> ()  [unwired: 2 out]
              }
            }
            n73 = Strip Path(path=w168) -> (stripped path=w166:path)  [unwired: 1 out]
            n74 = call-poly <userlib>:"Compare Two Paths__ogtk.vi"("path2"=w167, "path1"=w166) -> ("relative path from 1 to 2"=→"Path":path)  [unwired: 1 in, 2 out]
          }
          event "Listbox": Drag Starting? {
            n75 = event-data() -> ("CtlRef"=w200:refnum<vi>)  [unwired: 1 in]
            n76 = property class="LstBox (strict)"(reference=w200) -> ("Item Names"=w198:string[], "Value"=w197:i32)  [unwired: 1 in, 2 out]
            n77 = Index Array(array=w198, index=w197) -> (element=w196:string)
            n78 = Bundle(w195, w196) -> (w194:cluster{string, string})  [unwired: 1 in]
            n79 = Build Array(w194) -> (w193:cluster{string, string}[])
            n80 = Less Than 0?(x=w197) -> (x < 0?=w199:bool)
            n81 = event-data("Data"=w193, "Drag Mode"=enum32{"copy or move", "copy only", "move only"}."copy only", "Discard?"=w199) -> ()  [unwired: 1 in, 1 out]
          }
          event "Shift": Drop {
            # "/* Force Refresh */"
            n82 = event-data() -> ("CtlRef"=w209:refnum<vi>, "Available Data Names"=w212:string[])  [unwired: 1 in, 4 out]
            n83 = Search 1D Array(1D array=w212, element=w211) -> (index of element=w210:i32)  [unwired: 1 in]
            n84 = case shown="0.." w210 {
              tunnel: w211 -> [_ w221]
              tunnel: [_ TRUE] -> w208
              tunnel: w209 -> [_ _]
              tunnel: [_ w217] -> w207
              frame Default {
              }
              frame 0.. {
                n85 = Get Drag Drop Data(8:"" ("type"), 9:w221) -> (3:w218:string)  [unwired: 1 in, 1 out]
                n86 = call "TrimShortcutPrefix.vi"("String in"=w218) -> ("String out"=w217:string)  [unwired: 18 in]
              }
            }
            n87 = case shown="True" w208 {
              tunnel: w207 -> [_ w216]
              tunnel: w206 -> [_ w215]
              frame False {
              }
              frame True {
                n88 = call "ChangeAssignedShortcut.vi"("QDKS Info"=w215, "Key"="", "QD"=w216) -> ()  [unwired: 8 in, 1 out]
              }
            }
            n89 = event-data("Accepted?"=w208) -> ()  [unwired: 1 in, 1 out]
          }
          event "1", "2", "3", "4", "5", "6", "7", "8", "9", "0", "Q", "W", "E", "R", "T", "A", "S", "D", "F", "G", "Z", "X", "C", "V", "B", "Y", "U", "I", "O", "P", "H", "J", "K", "L", "N", "M", "Shift": Drag Enter {
            n90 = event-data() -> ("Available Data Names"=w229:string[])  [unwired: 1 in]
            n91 = Search 1D Array(1D array=w229, element=w228) -> (index of element=w227:i32)  [unwired: 1 in]
            n92 = Greater Or Equal To 0?(x=w227) -> (x >= 0?=w226:bool)
            n93 = event-data("Accepted?"=w226) -> ()  [unwired: 1 in, 1 out]
          }
          event "1", "2", "3", "4", "5", "6", "7", "8", "9", "0", "Q", "W", "E", "R", "T", "A", "S", "D", "F", "G", "Z", "X", "C", "V", "B", "Y", "U", "I", "O", "P", "H", "J", "K", "L", "N", "M": Drop {
            # "/* Force Refresh */"
            n94 = event-data() -> ("CtlRef"=w238:refnum<vi>, "Available Data Names"=w241:string[])  [unwired: 1 in, 4 out]
            n95 = Search 1D Array(1D array=w241, element=w240) -> (index of element=w239:i32)  [unwired: 1 in]
            n96 = case shown="0.." w239 {
              tunnel: w240 -> [_ w252]
              tunnel: [_ TRUE] -> w237
              tunnel: w238 -> [_ w247]
              tunnel: [_ w248] -> w235
              tunnel: [_ w246] -> w236
              frame Default {
              }
              frame 0.. {
                n97 = property class="Bool"(reference=w247) -> ("Label.Text"=w246:string)  [unwired: 1 in, 2 out]
                n98 = Get Drag Drop Data(8:"" ("type"), 9:w252) -> (3:w249:string)  [unwired: 1 in, 1 out]
                n99 = call "TrimShortcutPrefix.vi"("String in"=w249) -> ("String out"=w248:string)  [unwired: 18 in]
              }
            }
            n100 = case shown="True" w237 {
              tunnel: w236 -> [_ w244]
              tunnel: w235 -> [_ w245]
              tunnel: w234 -> [_ w243]
              frame False {
              }
              frame True {
                n101 = call "ChangeAssignedShortcut.vi"("QDKS Info"=w243, "Key"=w244, "QD"=w245) -> ()  [unwired: 8 in, 1 out]
              }
            }
            n102 = event-data("Accepted?"=w237) -> ()  [unwired: 1 in, 1 out]
          }
          event "[Trigger]Refresh Btns": Value Change {
            n103 = event-data() -> ()  [unwired: 1 in, 4 out]
            n104 = property class="VI"() -> (error out=w261:errorcluster, "Panel"=w260:refnum<vi>)  [unwired: 2 in, 1 out]
            n105 = property class="Pnl"(reference=w260, error in=w261, "DeferPanUpdts"=TRUE ("Defer Panel Updates")) -> (reference out=w259:refnum<vi>, error out=w258:errorcluster)
            n106 = property class="Pnl"(reference=w259, error in=w258) -> (reference out=w270:refnum<vi>, error out=w272:errorcluster, "AllObjs[]"=w271:refnum<vi>[])
            n107 = call "FilterBooleanRefs.vi"("error in (no error)"=w272, "AllObjs[]"=w271) -> ("error out"=w267:errorcluster, "AllObjs[] (dup)"=w268:refnum<vi>[])  [unwired: 8 in]
            n108 = disable-structure shown="Enabled" {
              disable-tunnel: w268 -> [w279 _]
              disable-tunnel: w256 -> [w278 _]
              disable-tunnel: w267 -> [w277 w280]
              disable-tunnel: [w276 w280] -> w265
              disable-tunnel: [w275 _] -> w266
              disable-tunnel: w254 -> [w274 _]
              frame Enabled {
                n109 = call "PopulateToBooleanRef.vi"("CounterMap"=w274, "QDKS Info"=w278, "error in (no error)"=w277, "AllObjs[]"=w279) -> ("error out"=w276:errorcluster, "AllObjs[] (dup)"=w275:refnum<vi>[])  [unwired: 6 in]
              }
              frame Disabled {
              }
            }
            n110 = call "UpdateBooleanRef.vi"("error in (no error)"=w265, "AllObjs[]"=w266) -> ("error out"=w264:errorcluster)  [unwired: 8 in, 1 out]
            n111 = Close Reference(reference=w271, error in (no error)=w264) -> (error out=w269:errorcluster)
            n112 = Close Reference(reference=w270, error in (no error)=w269) -> (error out=w263:errorcluster)
            n113 = property class="Pnl"(reference=w260, error in=w263, "DeferPanUpdts"=FALSE ("Defer Panel Updates")) -> ()  [unwired: 2 out]
          }
          event "[Trigger]Update QSDK Info": Value Change {
            n114 = event-data() -> ()  [unwired: 1 in, 6 out]
            n115 = call <resource>:"QuickDrop Get QDKS Info for Shortcut Dialog.vi"() -> ("QDKS Info"=w283:T2[])  [unwired: 11 in]
            n116 = for {
              tunnel: w283 -> [w312] mode=indexing
              tunnel: [w311] -> w293 mode=indexing
              n117 = Unbundle By Name(w312) -> ("VI Name"=w311:string)
            }
            n118 = call-poly <userlib>:"Remove Duplicates from 1D Array__ogtk.vi"("Input Array"=w293) -> ("Output Array"=w284:string[], "indices of removed elements"=w281:i32[])
            n119 = for {
              tunnel: w283 -> [w298] mode=indexing
              tunnel: [w298] -> w282 mode=indexing if=w294
              tunnel: w281 -> [w297]
              i -> [w296]
              n120 = Search 1D Array(1D array=w297, element=w296) -> (index of element=w295:i32)  [unwired: 1 in]
              n121 = Less Than 0?(x=w295) -> (x < 0?=w294:bool)
            }
            n122 = call <resource>:"LV Config Read String.vi"("default value"="", "key"="QuickDrop_NEVSTOP_LAST_EXECUTE") -> ("value"=w291:string)  [unwired: 3 in, 2 out]
            n123 = call-poly <userlib>:"Trim Whitespace__ogtk.vi"("String in"=w291) -> ("String out"=w292:string)  [unwired: 6 in]
            n124 = case shown="Default" w292 {
              selector: w292 -> [w308 _]
              tunnel: [w303 w309] -> w287
              tunnel: w282 -> [w307 w310]
              tunnel: [w300 w310] -> w288
              tunnel: w284 -> [w299 w309]
              frame Default {
                n125 = Search 1D Array(1D array=w299, element=w308) -> (index of element=w306:i32)  [unwired: 1 in]
                n126 = Delete From Array(array=w307, index=w306) -> (deleted portion=w301:T2, array with subset deleted=w302:T2[])  [unwired: 1 in]
                n127 = Delete From Array(array=w299, index=w306) -> (deleted portion=w305:string, array with subset deleted=w304:string[])  [unwired: 1 in]
                n128 = Build Array (concatenate)(w301, w302) -> (w300:T2[])
                n129 = Build Array (concatenate)(w305, w304) -> (w303:string[])
              }
              frame "" {
              }
            }
            n130 = call "LoadCounterCfg.vi"() -> ("Variant"=w286:variant)  [unwired: 11 in]
            "Variant" <- w286
          }
          event "Listbox": Mouse Down {
            n131 = event-data() -> ("CtlRef"=w315:refnum<vi>)  [unwired: 1 in]
            n132 = property class="LstBox (strict)"(reference=w315, "Key Focus"=FALSE) -> ()  [unwired: 1 in, 2 out]
          }
          event "[Trigger]Decorate List": Value Change {
            n133 = event-data() -> ()  [unwired: 1 in, 6 out]
            n134 = for {
              tunnel: w323 -> [w335] mode=indexing
              tunnel: [w328] -> w324 mode=indexing
              shift-right: [w329] -> w320
              shift-left: w321 -> [w332]
              n135 = Unbundle By Name(w335) -> ("VI Name"=w331:string, "Assigned Shortcut"=w334:string)
              n136 = Get Variant Attribute(Variant=w332, name=w331, default value (empty Variant)=0) -> (duplicate Variant=w329:variant, found=w326:bool, value=w327:i32)  [unwired: 1 in, 1 out]
              n137 = case shown="Default" w334 {
                selector: w334 -> [_ w343]
                tunnel: [_ w342] -> w333
                frame "" {
                }
                frame Default {
                  n138 = To Upper Case(1:w343) -> (0:w339:string)
                  n139 = Concatenate Strings("[" ("string"), w339, "] " ("string")) -> (w342:string)
                }
              }
              n140 = case shown="True" w326 {
                tunnel: w327 -> [_ w338]
                tunnel: [_ w336] -> w325
                frame False {
                }
                frame True {
                  n141 = Format Into String(format string="<%d> ", w338) -> (resulting string=w336:string)  [unwired: 2 in, 1 out]
                }
              }
              n142 = Concatenate Strings(w333, w325, w331) -> (w328:string)
            }
          }
        }
        n143 = case shown="False" w28 {
          tunnel: [w36 w39] -> w27
          tunnel: w26 -> [w37 w40]
          tunnel: w17 -> [_ w38]
          frame False {
            n144 = call "TrimShortcutPrefix.vi"("String in"=w37) -> ("String out"=w36:string)  [unwired: 18 in]
          }
          frame True {
            n145 = call "LookupQuickDrop.vi"("QDKS Info"=w38, "Key"=w40) -> ("QuickDrop"=w39:string)  [unwired: 8 in, 1 out]
          }
        }
        n146 = Not(x="Debug") -> (.not. x?=w29:bool)
        n147 = And(x=w29, y=w35) -> (x .and. y?=w31:bool)
      }
      n148 = call-poly <userlib>:"Trim Whitespace__ogtk.vi"("String in"=w12) -> ("String out"=w9:string)  [unwired: 6 in]
      n149 = case shown="False" w7 {
        tunnel: w9 -> [w15 _]
        tunnel: w8 -> [w14 _]
        frame False {
          n150 = call "UpdateCounterCfg.vi"("name"=w15, "Variant"=w14) -> ()  [unwired: 10 in]
        }
        frame True {
        }
      }
    }
    frame Error {
    }
  }
  "Cancelled?" <- w6
  "error out" <- w4
  "QuckDrop" <- w3
  "Shift Pressed" <- w2
  "QDKS Info" <- w1
  n151 = disable-structure shown="Disabled" {
    frame Disabled {
      n152 = property on="[Trigger]Refresh Btns" class="Bool (strict)"("Val(Sgnl)"=TRUE ("Value (Signaling)")) -> ()  [unwired: 2 in, 2 out]
      n153 = property on="[Trigger]Update QSDK Info" class="Bool (strict)"("Val(Sgnl)"=TRUE ("Value (Signaling)")) -> ()  [unwired: 2 in, 2 out]
      n154 = property on="Listbox" class="LstBox (strict)" props=["Val(Sgnl)"]() -> ()  [unwired: 3 in, 2 out]
      n155 = local read "Listbox"() -> ()  [unwired: 1 out]
      n156 = property on="Listbox" class="LstBox (strict)"("Top Row"=0) -> ()  [unwired: 2 in, 2 out]
    }
    frame Enabled {
    }
  }
